vi "SplineHelp_getQuinticSplinesFromControlVectors.vi"(11 "ControlVectors":T1[](array[typedef])) -> (0 "error out":errorcluster, 3 "splines":T2[](array[typedef]))   [LabVIEW 2019, in "Trajectory_Library.lvlib"]
doc: "Returns a set of quintic splines corresponding to the provided control vectors. The user is free to set the direction of all control vectors. Continuous curvature is guaranteed throughout the path.\n\nParameters:\n - controlVectors - The control vectors.\n\nReturns:\n - Splines - A vector of quintic hermite splines that interpolate through the provided waypoints.\n - Error Out - The returned error cluster"
uses:
  Trajectory_Library.lvlib
  SPLINE_CTRL_VECTOR.ctl
  <vilib>/Analysis/Matrix/Datatypes/RealMatrix.ctl
  <vilib>/Analysis/Matrix/NI_Matrix.lvlib
  SPLINE.ctl
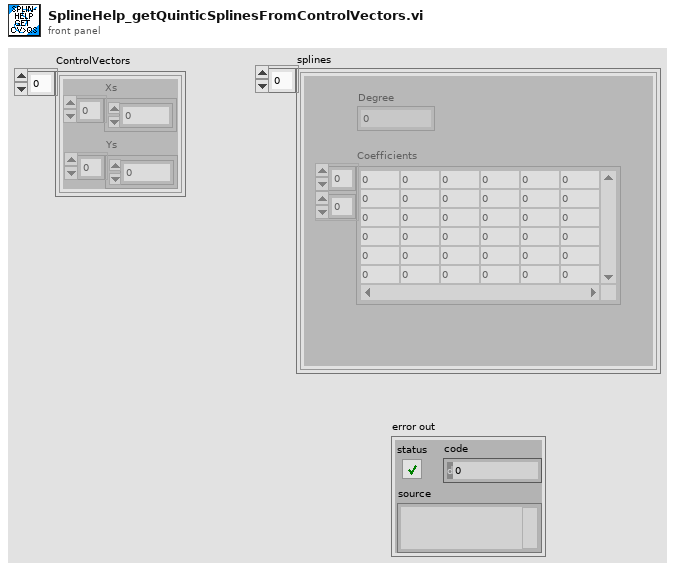
[diagram p1: front panel]
types:
  T1 = typedef "Trajectory_Library.lvlib/SPLINE_CTRL_VECTOR.ctl" = cluster{"Xs":dbl[], "Ys":dbl[]}
  T2 = typedef "Trajectory_Library.lvlib/SPLINE.ctl" = cluster{"Degree":i32, "Coefficients":T3}
  T3 = typedef "NI_Matrix.lvlib/RealMatrix.ctl" = dbl[][]
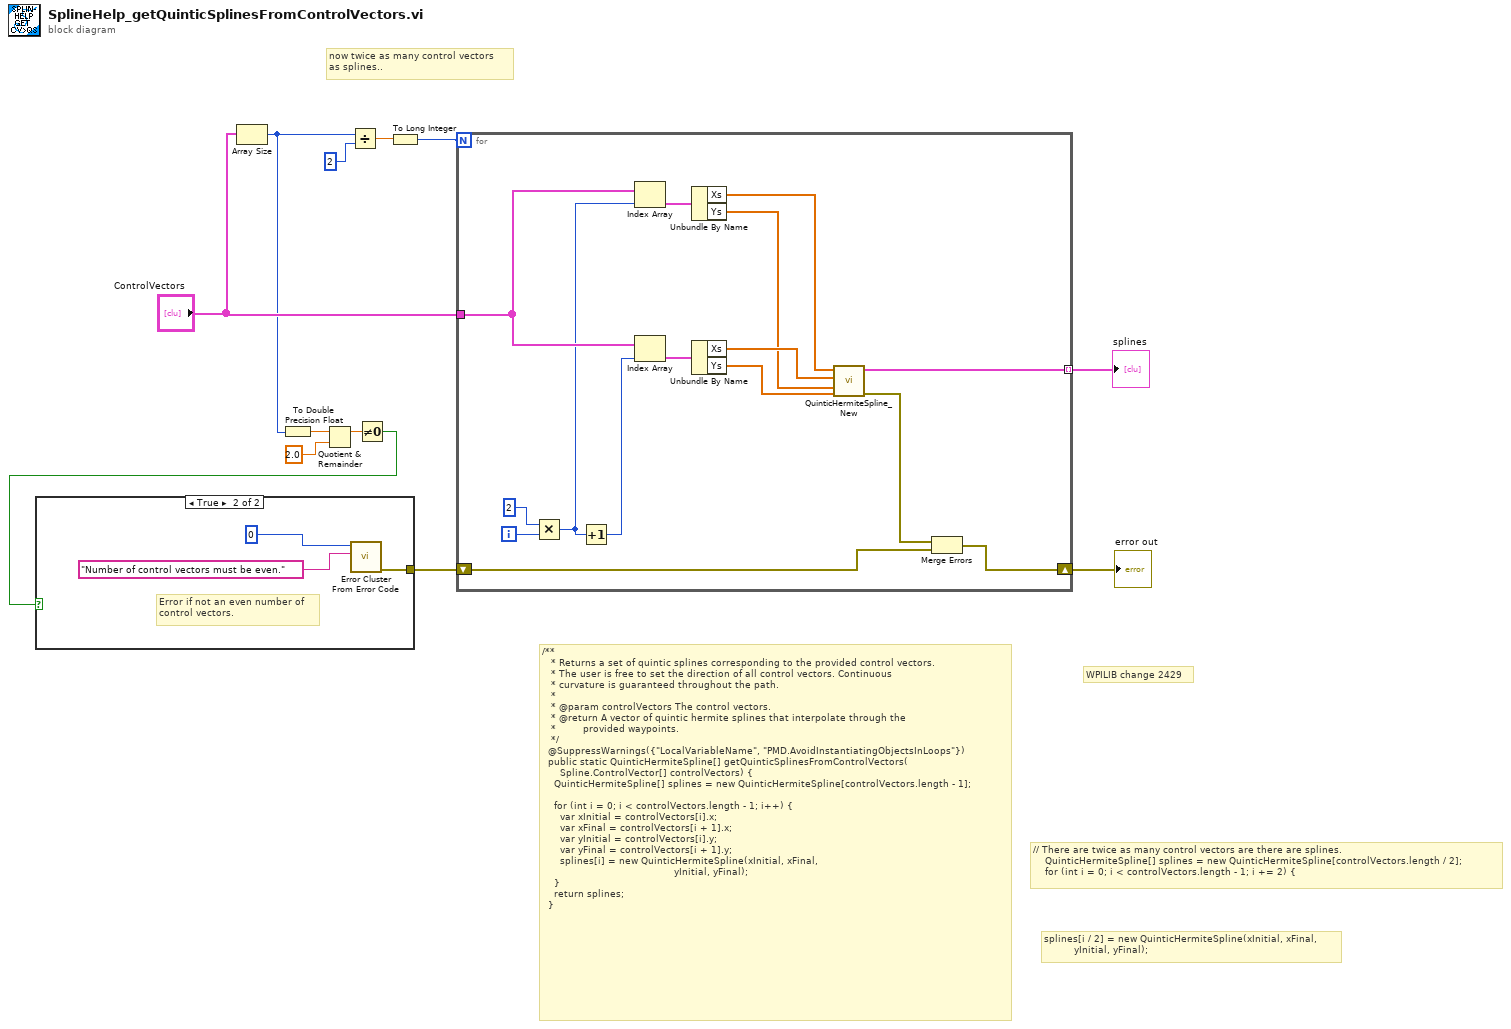
[diagram p0: block diagram]
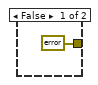
[diagram p2: hidden frame]
diagram:
  # "now twice as many control vectors\nas splines.."
  # "splines[i / 2] = new QuinticHermiteSpline(xInitial, xFinal,\n          yInitial, yFinal);"
  # "WPILIB change 2429"
  # "// There are twice as many control vectors are there are splines.\n    QuinticHermiteSpline[] splines = new QuinticHermiteSpline[controlVectors.length / 2];\n    for (int i = 0; i < controlVectors.length - 1; i += 2) {"
  # "/**\n   * Returns a set of quintic splines corresponding to the provided control vectors.\n   * The user is free to set the direction of all control vectors. Continuous\n   * curvature is guaranteed throughout the path.\n   *\n   * @param controlVectors The control vectors.\n   * @return A vector of quintic hermite splines that interpolate through the\n   *         provided waypoints.\n   */\n  @SuppressWarnings({\"LocalVariableName\", \"PMD.AvoidInstantiatingObjectsInLoops\"})\n  public static QuinticHermiteSpline[] getQuinticSplinesFromControlVectors(\n      Spline.ControlVector[] controlVectors) {\n    QuinticHermiteSpline[] splines = new QuinticHermiteSpline[controlVectors.length - 1];\n\n    for (int i = 0; i < controlVectors.length - 1; i++) {\n      var xInitial = controlVectors[i].x;\n      var xFinal = controlVectors[i + 1].x;\n      var yInitial = controlVectors[i].y;\n      var yFinal = controlVectors[i + 1].y;\n      splines[i] = new QuinticHermiteSpline(xInitial, xFinal,\n                                            yInitial, yFinal);\n    }\n    return splines;\n  }"
  n1 = Array Size(array="ControlVectors") -> (size(s)=w6:i32)
  n2 = To Double Precision Float(number=w6) -> (double precision float=w5:dbl)
  n3 = Quotient & Remainder(x=w5, y=2.0) -> (x-y*floor(x/y)=w3:dbl)  [unwired: 1 out]
  n4 = Divide(x=w6, y=2) -> (x/y=w8:dbl)
  n5 = Not Equal To 0?(x=w3) -> (x != 0?=w2:bool)
  n6 = case shown="True" w2 {
    tunnel: [errorcluster {"status"=FALSE, "code"=0, "source"=""} ("error out") w14] -> w1
    frame False {
    }
    frame True {
      # "Error if not an even number of\ncontrol vectors."
      n7 = call <vilib>:"Error Cluster From Error Code.vi"("error message (\"\")"="Number of control vectors must be even." ("error message (\"\")"), "error code (0)"=0) -> ("error out"=w14:errorcluster)  [unwired: 7 in]
    }
  }
  n8 = To Long Integer(number=w8) -> (32bit integer=w7:i32)
  n9 = for {
    N: w7 -> [_]
    tunnel: [w31] -> w12 mode=indexing
    shift-right: [w28] -> w11
    shift-left: w1 -> [w29]
    tunnel: "ControlVectors" -> [w26]
    i -> [w19]
    n10 = Multiply(x=2, y=w19) -> (x*y=w17:i32)
    n11 = Increment(x=w17) -> (x+1=w30:i32)
    n12 = Index Array(array=w26, index=w17) -> (element=w25:T1)
    n13 = Index Array(array=w26, index=w30) -> (element=w24:T1)
    n14 = Unbundle By Name(w25) -> ("Xs"=w23:dbl[], "Ys"=w21:dbl[])
    n15 = Unbundle By Name(w24) -> ("Xs"=w22:dbl[], "Ys"=w20:dbl[])
    n16 = call "QuinticHermiteSpline_New.vi"("yFinalCtrlVector"=w20, "yInitialCtrlVector"=w21, "xFinalCtrlVector"=w22, "XInitialCtrlVector"=w23) -> ("error out"=w27:errorcluster, "QuinticHermiteSpline"=w31:T2)  [unwired: 6 in]
    n17 = Merge Errors(w27, w29) -> (w28:errorcluster)
  }
  "error out" <- w11
  "splines" <- w12
